vi "Start Deploy.vi"(11 "FPGAtarget in":refnum<class "FPGATarget.lvclass">) -> (3 "FPGAtarget out":refnum<class "FPGATarget.lvclass">)   [LabVIEW 2020, in "NI_TargetHelper.lvlib" / "FPGATarget.lvclass"]
uses:
  <vilib>/TargetSupport/NI_TargetHelper/FPGATarget/FPGATarget.lvclass
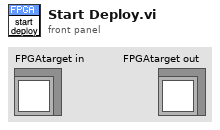
[diagram p1: front panel]
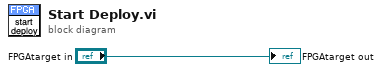
[diagram p0: block diagram]
diagram:
  "FPGAtarget out" <- "FPGAtarget in"
